vi "Remove Key Focus from VI.vi"(8 "error in (no error)":errorcluster, 11 "VI refnum":refnum<vi>) -> (0 "error out":errorcluster)   [LabVIEW 2017, in "NI_Robotics_Configure Steering Frame.lvlib"]
uses:
  <vilib>/robotics/Dialog/Configure Steering Frame/NI_Robotics_Configure Steering Frame.lvlib
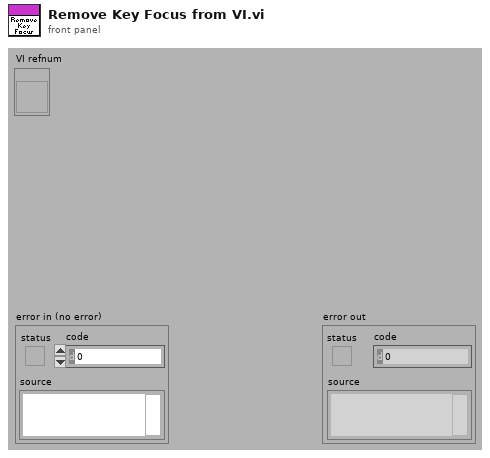
[diagram p1: front panel]
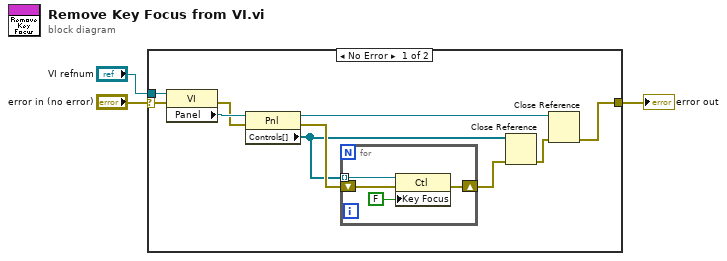
[diagram p0: block diagram]
diagram:
  n1 = case shown="No Error" "error in (no error)" {
    selector: "error in (no error)" -> [w4 w18]
    tunnel: "VI refnum" -> [w13 _]
    tunnel: [w5 w18] -> w2
    frame No Error {
      n2 = property class="VI"(reference=w13, error in=w4) -> (error out=w11:errorcluster, "Panel"=w12:refnum<vi>)  [unwired: 1 out]
      n3 = property class="Pnl"(reference=w12, error in=w11) -> (reference out=w6:refnum<vi>, error out=w10:errorcluster, "Controls[]"=w8:refnum<vi>[])
      n4 = for {
        tunnel: w8 -> [w17] mode=indexing
        shift-right: [w15] -> w9
        shift-left: w10 -> [w16]
        n5 = property class="Ctl"(reference=w17, error in=w16, "Key Focus"=FALSE) -> (error out=w15:errorcluster)  [unwired: 1 out]
      }
      n6 = Close Reference(reference=w8, error in (no error)=w9) -> (error out=w7:errorcluster)
      n7 = Close Reference(reference=w6, error in (no error)=w7) -> (error out=w5:errorcluster)
    }
    frame Error {
    }
  }
  "error out" <- w2
